vi "Analyze_Incorrect_Detections.vi"() -> ()   [LabVIEW 2020]
uses:
  <vilib>/Ngene/Deep Learning Toolkit/Toolkit/NN_Network/Controls/NN_Device.ctl
  <vilib>/Ngene/Deep Learning Toolkit/Toolkit/NN_Network/Controls/NN_Save_Before_Destroy_Options.ctl
  <vilib>/Ngene/Deep Learning Toolkit/Toolkit/NN_Data/API/Data/Detection_Types/NN_BBox_Detection.ctl
  <vilib>/Ngene/Deep Learning Toolkit/Toolkit/NN_Data/API/Data/Detection_Types/NN_BBox.ctl
  <vilib>/Utility/High Resolution Relative Seconds.vi
  <vilib>/Ngene/Deep Learning Toolkit/Toolkit/Utils/Vision/Coords_Rect2PolyLine.vi
  <vilib>/Ngene/Deep Learning Toolkit/Toolkit/NN_Network/subVIs/NN_Predict/NN_Predict(In3D_OutBBox).vi
  <vilib>/Ngene/Deep Learning Toolkit/Toolkit/NN_Train/Eval_Loss/NN_Eval_Test_Error_Loss/NN_Eval(In3D_OutBBox).vi
  <vilib>/Ngene/Deep Learning Toolkit/Toolkit/Deep_Learning_Toolkit_by_Ngene.lvlib
panel:
  in  "Class_Idx":i32
  out "Labels":string[](array[string])=["Nut", "Screw", "Washer"]
  out "All GTs":i32=456
  out "All Preds":i32=443
  out "FP Count":i32=2
  out "FN Count":i32=15
  out "Recall":dbl=0.9671052631578947
  out "Precision":dbl=0.9954853273137697
  out "mIOU":sgl=0.8432986 format="%0.2f"
  out "mAP":sgl=0.9881089 format="%0.2f"
  out "# of False Imgs":i32=13
  out "DS_Size":i32=74
  in  "TP_IOU_thresh":sgl=0.41
  in  "mBatch":i32=16
  in  "Dataset Path (Annotations)":path=path "D:/DNN/Nuts_Bolts/2023_07_26/00_orig_Fixed v2/test/Annotations"
  in  "Dataset Path (Images)":path=path "D:/DNN/Nuts_Bolts/2023_07_26/00_orig_Fixed v2/test/Images"
  in  "NMS_IOU_Thrsh":sgl=0.2
  in  "Confidence_Thrsh":sgl=0.5
  in  "NN_Device":T1=enum."GPU"
  in  "Trained Model Weights":path=path "D:/Ngene/Projects_SVN/DeepLTK/Examples/3_Image_Processing/3_3_Object_Detection/_GitHUB/3_3_Object_Detection/Models/Fixed_DS_v2_Aud(4x)_Dims_In_512x910/Obj_Det_Example_weights_25_06_04__18_09_23.bin"
  in  "Model Topology":path=path "D:/Ngene/Projects_SVN/DeepLTK/Examples/3_Image_Processing/3_3_Object_Detection/_GitHUB/3_3_Object_Detection/Models/Fixed_DS_v2_Aud(4x)_Dims_In_512x910/Obj_Det_Example_net_cfg_25_06_04__18_09_23.cfg"
  in  "Stop":bool
  out "Image":T2(plugin-control)
  in  "Select Sample":i32=5 min=0 max=37 step=1
  out "Sample Path":path
  in  "Preds Color":u32[](array[colorbox])=[16711686, 15679744, 16711680, 1740031, 13311, 33023, 52479, 65509, 65433, 65356, 65280, 5111552, 10092288, 15138560, 16763904, 16744192, 16724736, 16711680, 16711680, 16711680]
  in  "GT Color":u32[](array[colorbox])=[6618880, 6618880, 6618880, 1740031, 13311, 33023, 52479, 65509, 65433, 65356, 65280, 5111552, 10092288, 15138560, 16763904, 16744192, 16724736, 16711680, 16711680, 16711680]
  in  "fontsize":sgl=9.0
  out "FNs":cluster{"Array":bool[]}={"Array"=[FALSE, TRUE, TRUE, TRUE, TRUE, FALSE, FALSE]}
  out "FPs":cluster{"Array":bool[]}={"Array"=[TRUE, TRUE, TRUE, TRUE]}
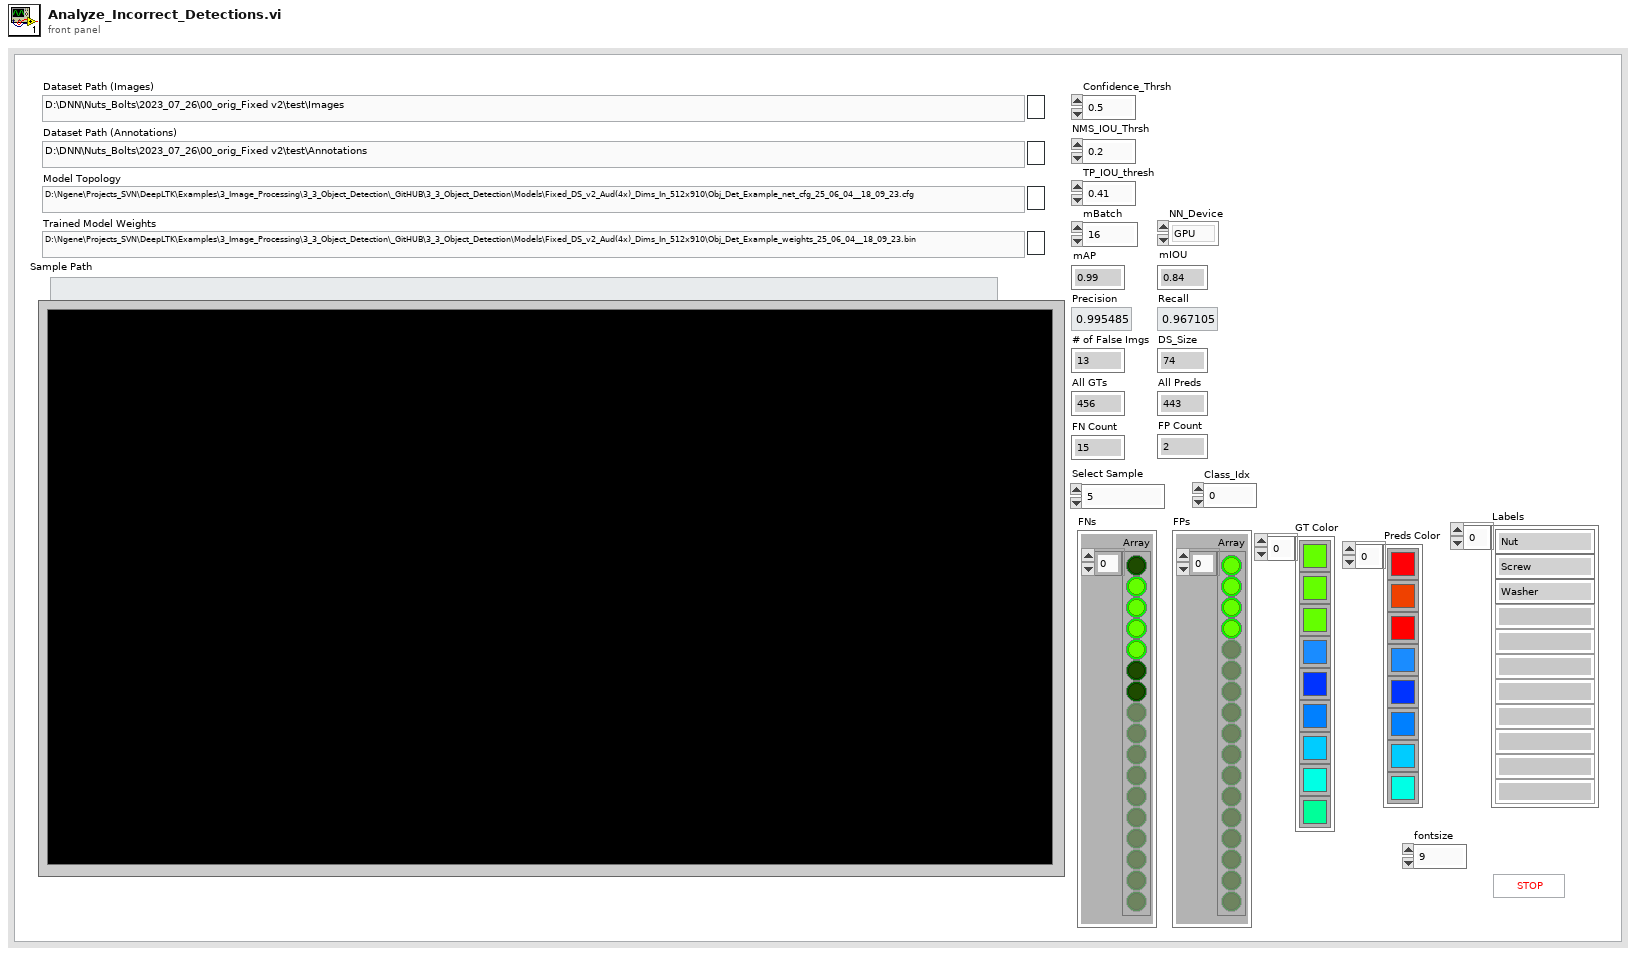
[diagram p1: front panel]
types:
  T1 = typedef "Deep_Learning_Toolkit_by_Ngene.lvlib/NN_Device.ctl" = enum16{"CPU", "GPU"}
  T2 = typedef "IMAQ Image.ctl" = refnum<image>
  T3 = typedef "Image Type" = u32
  T4 = typedef "Deep_Learning_Toolkit_by_Ngene.lvlib/NN_Save_Before_Destroy_Options.ctl" = cluster{"CFG?":bool, "Weights?":bool, "Render?":bool}
  T5 = typedef "Deep_Learning_Toolkit_by_Ngene.lvlib/NN_Config_Params.ctl" = cluster{"Name":string, "mBatch":i32, "NN_Train_Params":T6, "LR_Decay_Policy":T9, "Labels":string[], "Loss":T11, "Max_WS_Size(B)":i64, "DryRun?":bool}
  T6 = typedef "Deep_Learning_Toolkit_by_Ngene.lvlib/NN_Train_Params.ctl" = cluster{"Optimizer":T7, "Beta_1":sgl, "Beta_2":sgl, "Weight Decay(L1)":sgl, "Weight Decay(L2)":sgl, "Data_Sampling":T8}
  T7 = typedef "Deep_Learning_Toolkit_by_Ngene.lvlib/NN_Train_Optimizer.ctl" = enum16{"SGD", "Adam", "Adagrad", "Adadelta", "RMSProp", "Nesterov"}
  T8 = typedef "Deep_Learning_Toolkit_by_Ngene.lvlib/NN_Train_Data_Sampling.ctl" = enum16{"Random", "Sequential"}
  T9 = typedef "Deep_Learning_Toolkit_by_Ngene.lvlib/NN_LR_Policy_Cfg.ctl" = cluster{"Policy_Type":T10, "LR0":dbl, "k":sgl, "WarmUp_Policy":enum16{"Step", "Ramp"}, "WarmUp_Iter":i32, "WarmUp_Ratio":sgl}
  T10 = typedef "Deep_Learning_Toolkit_by_Ngene.lvlib/NN_LR_Policy_Type.ctl" = enum16{"Manual", "Step", "Exp", "1/t"}
  T11 = typedef "Deep_Learning_Toolkit_by_Ngene.lvlib/NN_Loss_Config_Params.ctl" = cluster{"Loss_Type":T12, "Loss_Conf_Params":variant}
  T12 = typedef "Deep_Learning_Toolkit_by_Ngene.lvlib/NN_Loss_Type.ctl" = enum16{"None", "MSE", "CrossEntropy", "YOLO_v2", "YOLO_v4"}
  T13 = typedef "Deep_Learning_Toolkit_by_Ngene.lvlib/NN_Layer_Config_Params.ctl" = cluster{"Layer_Type":T14, "Layer_Conf_Params":variant, "Input Layers":string[]}
  T14 = typedef "Deep_Learning_Toolkit_by_Ngene.lvlib/NN_Layer_Type.ctl" = enum16{"Input1D", "Input3D", "Conv1D", "Conv2D", "Conv2D_Adv", "MaxPool", "AvgPool", "UpSample", "DropOut3D", "ShortCut", "Concat", "SoftMax3D", "FC", "DropOut", "Softmax", "Flatten", "YOLO_v2", "YOLO_v4", "Activation", "BatchNormalization", "LayerNormalization", "Scale", "Unsupported"}
  T15 = typedef "Deep_Learning_Toolkit_by_Ngene.lvlib/NN.ctl" = cluster{"Name":string, "No of Layers":i32, "mBatch":i32, "Layers":T16[], "Dimty":T17, "Dims_In":T18, "Dims_Out":T18, "Working_Dir":path, "Train?":bool, "Train_Params":T6, "LR_Update_Policy":T9, "Session Data":T19, "Ground_truth":T20, "NNg_hdls":T21, "NN_Device":T1, "GPU Id":i32, "Labels":string[], "Loss_Type":T12, "Loss_Cfg_Prms":variant, "NNG_WS":T22, "DryRun?":bool}
  T16 = typedef "Deep_Learning_Toolkit_by_Ngene.lvlib/NN_Layer_ref.ctl" = refnum<file>
  T17 = typedef "Deep_Learning_Toolkit_by_Ngene.lvlib/NN_In_Out_Dim-ty.ctl" = enum8{"In1D_Out1D", "In3D_Out1D", "In3D_Out3D", "In3D_OutBBox"}
  T18 = typedef "Deep_Learning_Toolkit_by_Ngene.lvlib/NN_Dims(C,H,W).ctl" = cluster{"C":i32, "H":i32, "W":i32}
  T19 = typedef "Deep_Learning_Toolkit_by_Ngene.lvlib/NN_Train_Session_Data.ctl" = cluster{"Epochs":sgl, "Tot_Iter":i32, "LR":sgl, "LR_iter":i32}
  T20 = typedef "Deep_Learning_Toolkit_by_Ngene.lvlib/NN_Ground_truth.ctl" = cluster{"Y":variant}
  T21 = typedef "Deep_Learning_Toolkit_by_Ngene.lvlib/nng_cuda_handles.ctl" = cluster{"cudnn":u64, "cublas":u64, "stream":u64, "curand":u64}
  T22 = typedef "Deep_Learning_Toolkit_by_Ngene.lvlib/NNG_WS.ctl" = cluster{"NNG_WS_Mem":T23, "Max_WS_Size":i64}
  T23 = typedef "Deep_Learning_Toolkit_by_Ngene.lvlib/NNg_WS_Mem_DVR.ctl" = refnum<data-value>
  T24 = typedef "Deep_Learning_Toolkit_by_Ngene.lvlib/NN_DataSets_All(In3D_OutBBox).ctl" = cluster{"Train":T25, "Validation":T25, "Test":T25}
  T25 = typedef "Deep_Learning_Toolkit_by_Ngene.lvlib/NN_DataSet(In3D_OutBBox).ctl" = cluster{"Inputs Ref.":variant, "Dataset_Size":i32, "Dims_In":T18, "Outputs Refs":T26, "No of Classes ":i32, "Labels":string[], "File Paths":path[], "Custom_Data":variant}
  T26 = typedef "Deep_Learning_Toolkit_by_Ngene.lvlib/NN_Data_ref(1D_BBox).ctl" = refnum<data-value>
  T27 = typedef "Deep_Learning_Toolkit_by_Ngene.lvlib/NN_Image_Detections.ctl" = cluster{"Image Detections":T28[]}
  T28 = typedef "Deep_Learning_Toolkit_by_Ngene.lvlib/NN_BBox_Detection.ctl" = cluster{"Class":i32, "Conf Level":sgl, "BBox":T29}
  T29 = typedef "Deep_Learning_Toolkit_by_Ngene.lvlib/NN_BBox.ctl" = cluster{"x":sgl, "y":sgl, "w":sgl, "h":sgl}
  T30 = typedef "Deep_Learning_Toolkit_by_Ngene.lvlib/NN_Image_Annotations.ctl" = cluster{"Image Annotations":T31[]}
  T31 = typedef "Deep_Learning_Toolkit_by_Ngene.lvlib/NN_BBox_Annotation.ctl" = cluster{"Class":i32, "BBox":T29}
  T32 = typedef "Deep_Learning_Toolkit_by_Ngene.lvlib/NN_Eval_Params(in3D_OutBBox).ctl" = cluster{"Precision@Max_Avg_F1_Score":sgl, "Recall@Max_Avg_F1_Score":sgl, "argmax_avgF1_Score(Conf)":sgl, "Max_Avg_F1_Score":sgl, "Max_F1_Score_Per_Class":sgl[], "F1_Score_Per_Class":sgl[][], "Avg_F1,P,R Curves":cluster{"Conf":sgl[], "F1|P|R":sgl[]}[], "mIOU":sgl, "APs@0.5":sgl[], "PR_Curves@0.5":T33, "IOUs":sgl[], "mAP@0.75":sgl, "mAP@0.5-0.95":sgl, "mAP@0.5":sgl, "Mean_PR_Curve":T34}
  T33 = typedef "Deep_Learning_Toolkit_by_Ngene.lvlib/NN_PR_Curves.ctl" = T34[]
  T34 = typedef "Deep_Learning_Toolkit_by_Ngene.lvlib/NN_PR.ctl" = cluster{"Recall":sgl[], "Precision":sgl[]}
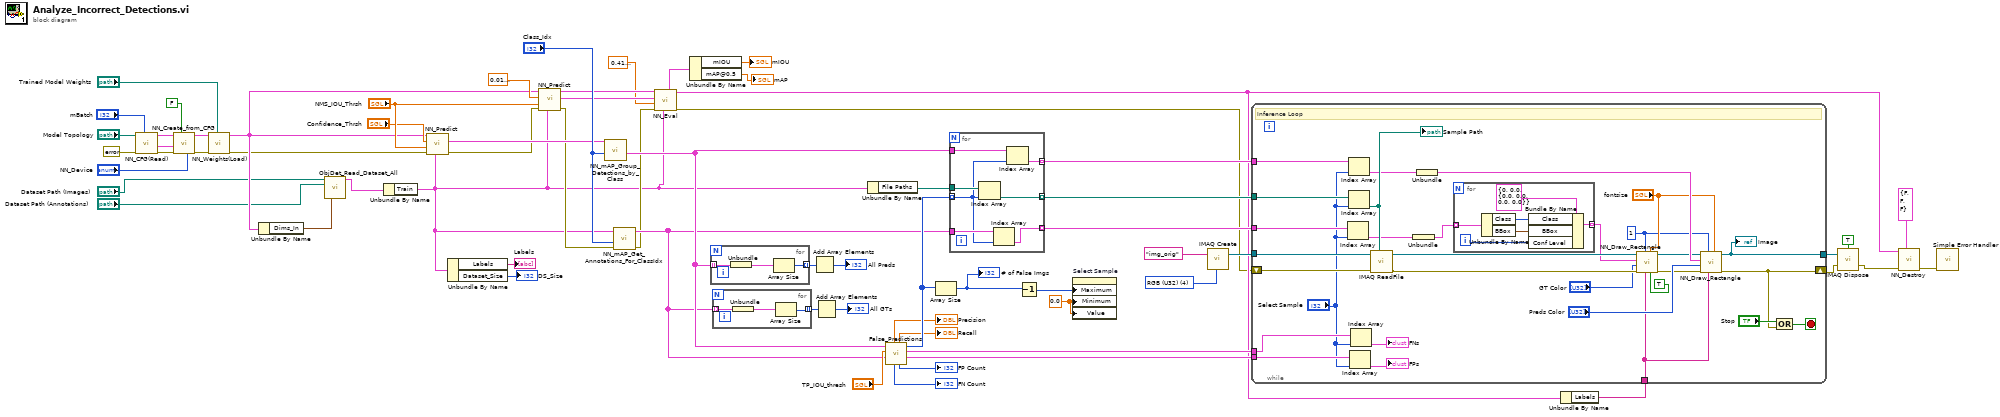
[diagram p0: block diagram]
diagram:
  w39 = 0.0 ("Data Entry Limits:Minimum")
  w49 = T3 4 items=["Grayscale (U8)", "Grayscale (I16)", "Grayscale (SGL)", "Complex (CSG)", "RGB (U32)", "HSL (U32)", "RGB (U64)", "Grayscale (U16)"] ("Image Type")
  n1 = call <vilib>:"NN_CFG(Read).vi"("mBatch"="mBatch", "error in (no error)"=errorcluster {"status"=FALSE, "code"=0, "source"=""}, "CFG file path"="Model Topology") -> ("error out"=w65:errorcluster, "Net_Cfg"=w61:T5, "Layer_Cfg"=w66:T13[])  [unwired: 6 in]
  n2 = call <vilib>:"NN_Create_from_CFG.vi"("NN_Device"="NN_Device", "Train? (false)"=FALSE, "error in (no error)"=w65, "Net_Cfg"=w61, "Layer_Cfg"=w66) -> ("error out"=w64:errorcluster, "NN out"=w62:T15)  [unwired: 5 in]
  n3 = call <vilib>:"NN_Weights(Load).vi"("Weight File Path"="Trained Model Weights", "error in (no error)"=w64, "NN in"=w62) -> ("error out"=w5:errorcluster, "NN out"=w8:T15)  [unwired: 7 in]
  n4 = Unbundle By Name(w8) -> ("Dims_In"=w7:T18)
  n5 = call "ObjDet_Read_Dataset_All.vi"("Train Image Path"="Dataset Path (Images)", "Train Anno Path"="Dataset Path (Annotations)", "Dims(C,H,W)"=w7) -> ("Dataset"=w6:T24)  [unwired: 10 in, 2 out]
  n6 = Unbundle By Name(w6) -> ("Train"=w4:T25)
  n7 = call-poly <vilib>:"NN_Predict.vi"("Dataset"=w4, "error in (no error)"=w5, "NMS_IOU_Thresh(0.5)"="NMS_IOU_Thrsh", "Conf_Thresh(0.5)"="Confidence_Thrsh", "NN in"=w8) -> ("error out"=w25:errorcluster, "Predictions"=w40:T27[])  [unwired: 4 in, 1 out]
  n8 = Unbundle By Name(w4) -> ("Labels"=→"Labels":string[], "Dataset_Size"=→"DS_Size":i32)
  n9 = call-poly <vilib>:"NN_Predict.vi"("Dataset"=w4, "error in (no error)"=w25, "NMS_IOU_Thresh(0.5)"="NMS_IOU_Thrsh", "Conf_Thresh(0.5)"=sgl 0.02, "NN in"=w8) -> ("error out"=w20:errorcluster, "Predictions"=w10:T27[], "NN out"=w24:T15)  [unwired: 4 in]
  n10 = call <vilib>:"NN_mAP_Group_Detections_by_Class.vi"("Class_Idx"="Class_Idx", "Detections(in Dataset)"=w40) -> ("Detections_for_ClassIdx(by_Image)"=w34:T27[])  [unwired: 7 in, 2 out]
  n11 = call <vilib>:"NN_mAP_Get_Annotations_For_ClassIdx.vi"("error in (no error)"=w20, "Class_Idx"="Class_Idx", "Dataset_Refs"=w4) -> ("error out"=w19:errorcluster, "Annotations_for_ClassIdx"=w26:T30[])  [unwired: 7 in]
  n12 = call-poly <vilib>:"NN_Eval.vi"("Dataset"=w4, "error in"=w19, "IOU_Conf_Thrsh(0.5)"=sgl 0.42, "Detections(in Dataset)"=w10, "NN in"=w24) -> ("error out"=w16:errorcluster, "NN out"=w18:T15, "NN_Eval_Params"=w13:T32)  [unwired: 4 in]
  n13 = Unbundle By Name(w13) -> ("mIOU"=→"mIOU":sgl, "mAP@0.5"=→"mAP":sgl)
  n14 = for {
    tunnel: w34 -> [w70] mode=indexing
    tunnel: [w68] -> w32 mode=indexing
    n15 = Unbundle(w70) -> ("Image Detections"=w69:T28[])
    n16 = Array Size(array=w69) -> (size(s)=w68:i32)
  }
  n17 = for {
    tunnel: w26 -> [w73] mode=indexing
    tunnel: [w71] -> w28 mode=indexing
    n18 = Unbundle(w73) -> ("Image Annotations"=w72:T31[])
    n19 = Array Size(array=w72) -> (size(s)=w71:i32)
  }
  n20 = Add Array Elements(numeric array=w32) -> (sum=→"All Preds":i32)
  n21 = Add Array Elements(numeric array=w28) -> (sum=→"All GTs":i32)
  n22 = Unbundle By Name(w4) -> ("File Paths"=w54:path[])
  n23 = call "False_Predictions.vi"("Annotations_for_ClassIdx"=w26, "TP_IOU_thresh"="TP_IOU_thresh", "Detections_for_ClassIdx(by_Image)"=w34) -> ("FPs"=w35:cluster{"Array":bool[]}[], "FNs"=w36:cluster{"Array":bool[]}[], "Incorrect classified samples"=w43:i32[], "#FP"=→"FP Count":i32, "Recall"=→"Recall":dbl, "#FN"=→"FN Count":i32, "Precision"=→"Precision":dbl)  [unwired: 1 in, 1 out]
  n24 = Array Size(array=w43) -> (size(s)=w42:i32)
  "# of False Imgs" <- w42
  n25 = for {
    tunnel: w54 -> [w80]
    tunnel: w43 -> [w76] mode=indexing
    tunnel: [w79] -> w48 mode=indexing
    tunnel: w34 -> [w78]
    tunnel: w26 -> [w77]
    tunnel: [w75] -> w47 mode=indexing
    tunnel: [w74] -> w46 mode=indexing
    n26 = Index Array(array=w80, index=w76) -> (element=w79:path)
    n27 = Index Array(array=w77, index=w76) -> (element=w74:T30)
    n28 = Index Array(array=w78, index=w76) -> (element=w75:T27)
  }
  n29 = Decrement(x=w42) -> (x-1=w41:i32)
  n30 = property on="Select Sample" class="DigNum (strict)"("Maximum"=w41, "Minimum"=w39, "Value"=w39) -> ()  [unwired: 2 in, 2 out]
  n31 = call "IMAQ Create"("Image Name"="img_orig", "Image Type"=w49) -> ("New Image"=w50:T2)  [unwired: 3 in, 1 out]
  n32 = Unbundle By Name(w18) -> ("Labels"=w45:string[])
  n33 = while {
    tunnel: [w105] -> w53
    tunnel: w48 -> [w108]
    tunnel: w50 -> [w107]
    shift-right: [w103] -> w15
    shift-left: w16 -> [w106]
    tunnel: w47 -> [w102]
    tunnel: w46 -> [w101]
    tunnel: w45 -> [w90]
    tunnel: w36 -> [w87]
    tunnel: w35 -> [w86]
    stop <- w109 stop-if-true
    w88 = u32 1 ("Border_Width")
    # "Inference Loop"
    n34 = Index Array(array=w101, index="Select Sample") -> (element=w98:T30)
    n35 = Index Array(array=w102, index="Select Sample") -> (element=w100:T27)
    n36 = Index Array(array=w108, index="Select Sample") -> (element=w104:path)
    "Sample Path" <- w104
    n37 = Index Array(array=w86, index="Select Sample") -> (element=→"FPs":cluster{"Array":bool[]})
    n38 = Index Array(array=w87, index="Select Sample") -> (element=→"FNs":cluster{"Array":bool[]})
    n39 = call "IMAQ ReadFile"("File Path"=w104, "error in (no error)"=w106, "Image"=w107) -> ("error out"=w95:errorcluster, "Image Out"=w94:T2)  [unwired: 4 in, 3 out]
    n40 = Unbundle(w98) -> ("Image Annotations"=w97:T31[])
    n41 = Unbundle(w100) -> ("Image Detections"=w96:T28[])
    n42 = for {
      tunnel: w97 -> [w114] mode=indexing
      tunnel: [w115] -> w91 mode=indexing
      i -> [w111]
      n43 = Unbundle By Name(w114) -> ("Class"=w113:i32, "BBox"=w112:T29)
      n44 = Bundle By Name(cluster=T28 {"Class"=0, "Conf Level"=0.0, "BBox"={"x"=0.0, "y"=0.0, "w"=0.0, "h"=0.0}} ("Image Detections"), "Class"=w113, "BBox"=w112, "Conf Level"=w111) -> (w115:T28)
    }
    n45 = call "NN_Draw_Rectangle.vi"("Clear Overlays?"=TRUE ("Clear"), "font_size"="fontsize", "Labels"=w90, "Border_Width"=w88, "error in (no error)"=w95, "Colors"="GT Color", "Draw_Boxes"=w91, "Img in"=w94) -> ("error out"=w92:errorcluster, "Img out"=w93:T2)  [unwired: 2 in]
    n46 = call "NN_Draw_Rectangle.vi"("font_size"="fontsize", "Labels"=w90, "Border_Width"=w88, "error in (no error)"=w92, "Colors"="Preds Color", "Draw_Boxes"=w96, "Img in"=w93) -> ("error out"=w103:errorcluster, "Img out"=w105:T2)  [unwired: 3 in]
    "Image" <- w105
    n47 = Compound Arithmetic op=OR("Stop", w103) -> (w109:bool)
  }
  n48 = call "IMAQ Dispose"("All Images? (No)"=TRUE, "Image"=w53, "error in (no error)"=w15) -> ("error out"=w14:errorcluster)  [unwired: 3 in]
  n49 = call <vilib>:"NN_Destroy.vi"("Save (T, T, T)"=T4 {"CFG?"=FALSE, "Weights?"=FALSE, "Render?"=FALSE}, "error in (no error)"=w14, "NN in"=w18) -> ("error out"=w17:errorcluster)  [unwired: 7 in, 1 out]
  n50 = call <vilib>:"Simple Error Handler.vi"("error in (no error)"=w17) -> ()  [unwired: 4 in, 5 out]
